vi "Request current CH2 (SubVI).vi"() -> (3 "Request current CH2 / Y":string)   [LabVIEW 2018]
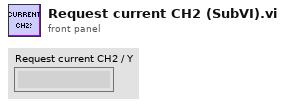
[diagram p1: front panel]
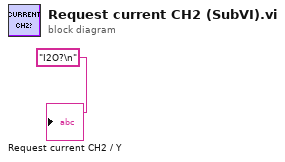
[diagram p0: block diagram]
diagram:
  "Request current CH2 / Y" <- "I2O?\n" ("format string")
